vi "INI.Content to Attributes.vi"(10 "Content":string, 11 "Section Name":string) -> (2 "Section Attributes":variant)   [LabVIEW 2013, in "OpenSerializer.lvlib" / "Serializer.PlainText.INI.lvclass"]
doc: "JKI SMO Configuration 1.2.1.18\nJKI - JKI\nCopyright (c) 2017, JKI"
uses:
  Serializer.PlainText.INI.lvclass
  <vilib>/regexp/Match Regular Expression.xnode
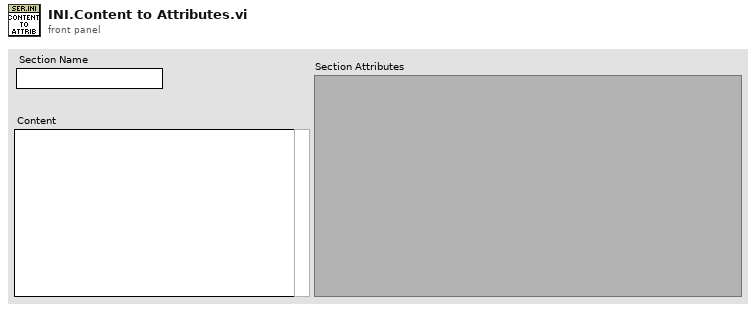
[diagram p1: front panel]
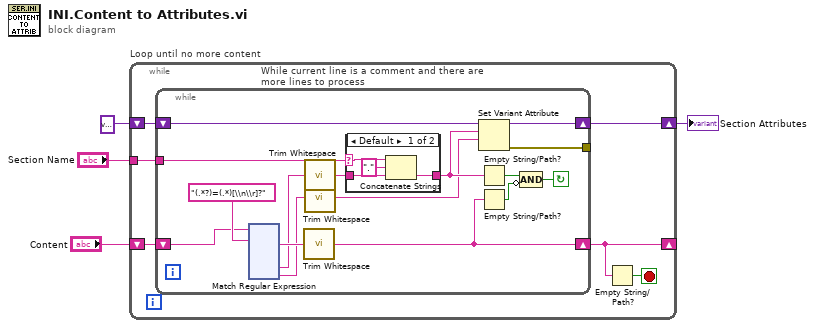
[diagram p0: block diagram]
diagram:
  n1 = while "Loop until no more content" {
    shift-right: [w7] -> w4
    shift-left: variant -> [w8]
    shift-right: [w6] -> _
    shift-left: "Content" -> [w10]
    tunnel: "Section Name" -> [w5]
    stop <- w9 stop-if-true
    n2 = while "While current line is a comment and there are more lines to process" {
      shift-right: [w23] -> w6
      shift-left: w10 -> [w16]
      shift-right: [w21] -> w7
      shift-left: w8 -> [w22]
      tunnel: [w20] -> _
      tunnel: w5 -> [w19]
      stop <- w24 continue-if-true
      n3 = xnode "Match Regular Expression"("input string"=w16, "regular expression"="(.*?)=(.*)[\\n\\r]?") -> ("after match"=w15:string, "submatch 1"=w14:string, "submatch 2"=w12:string)  [unwired: 4 in, 4 out]
      n4 = call <vilib>:"Trim Whitespace.vi"("string"=w15) -> ("trimmed string"=w23:string)  [unwired: 1 in]
      n5 = call <vilib>:"Trim Whitespace.vi"("string"=w14) -> ("trimmed string"=w13:string)  [unwired: 1 in]
      n6 = call <vilib>:"Trim Whitespace.vi"("string"=w12) -> ("trimmed string"=w11:string)  [unwired: 1 in]
      n7 = case shown="Default" w19 {
        selector: w19 -> [w146 _]
        tunnel: w13 -> [w145 w148]
        tunnel: [w147 w148] -> w18
        frame Default {
          n8 = Concatenate Strings(w146, "." ("string"), w145) -> (w147:string)
        }
        frame "" {
        }
      }
      n9 = Set Variant Attribute(Variant=w22, name=w18, value=w11) -> (Variant out=w21:variant, error out=w20:errorcluster)  [unwired: 1 in, 1 out]
      n10 = Empty String/Path?(string/path=w18) -> (empty?=w26:bool)
      n11 = Empty String/Path?(string/path=w23) -> (empty?=w25:bool)
      n12 = Compound Arithmetic op=AND(w26, invert w25) -> (w24:bool)
    }
    n13 = Empty String/Path?(string/path=w6) -> (empty?=w9:bool)
  }
  "Section Attributes" <- w4
